vi "Intake Limit Safety.vi"(10 "Motor Power":dbl, 11 "Wrist up?":bool) -> (3 "Motor Out":dbl)   [LabVIEW 2017]
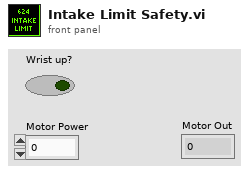
[diagram p1: front panel]
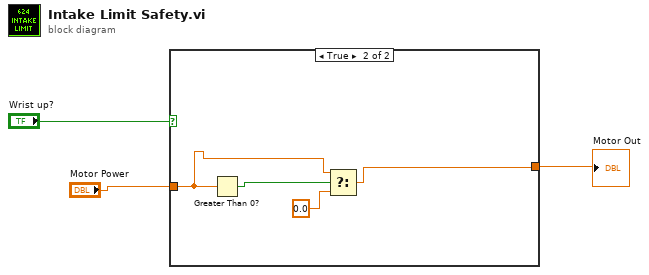
[diagram p0: block diagram]
diagram:
  n1 = case shown="True" "Wrist up?" {
    tunnel: "Motor Power" -> [w4 w7]
    tunnel: [w4 w5] -> w1
    frame False {
    }
    frame True {
      n2 = Greater Than 0?(x=w7) -> (x > 0?=w8:bool)
      n3 = Select(t=w7, s=w8, f=0.0) -> (s? t:f=w5:dbl)
    }
  }
  "Motor Out" <- w1
